vi "WPI_AnalogModuleOpen.vi"(8 "error in (no error)":errorcluster) -> (0 "error out":errorcluster, 3 "AnalogModuleDevRef":T1)   [LabVIEW 2017]
doc: "This software is licensed. Open the labview\\readme\\WPI Robotics Library Open Source License.txt file for more information."
uses:
  <vilib>/Rock Robotics/WPI/AnalogModule/WPI_AnalogModuleDevStatus.ctl
  <vilib>/Rock Robotics/SystemInterfaces/AI/FPGA_AIChannel.ctl
  <vilib>/Rock Robotics/SystemInterfaces/System/FPGA_SystemGet.vi
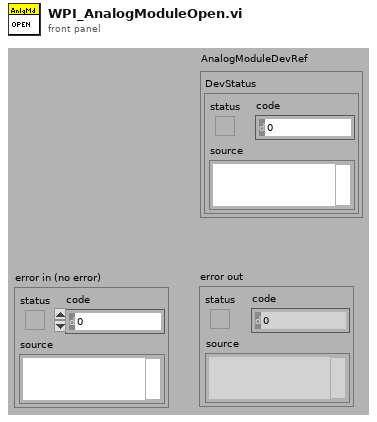
[diagram p1: front panel]
types:
  T1 = typedef "WPI_AnalogModuleDevStatus.ctl" = cluster{"DevStatus":errorcluster}
  T2 = typedef "FPGA_AIDevRef.ctl" = cluster{"DevStatus":errorcluster}
  T3 = typedef "FPGA_AIChannel.ctl" = enum8{"AI 0", "AI 1", "AI 2", "AI 3", "AI MXP 0", "AI MXP 1", "AI MXP 2", "AI MXP 3", "Invalid"}
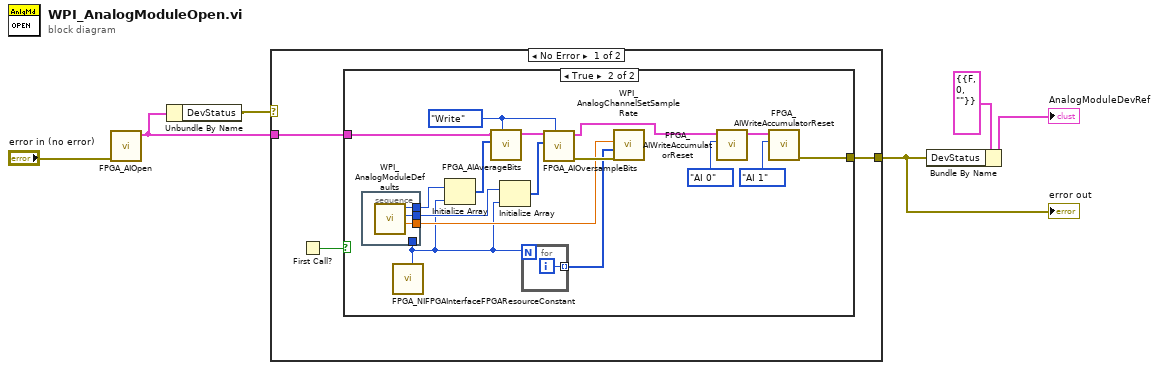
[diagram p0: block diagram]
diagram:
  n1 = call <vilib>:"FPGA_AIOpen.vi"("error in (no error)"="error in (no error)") -> ("AI Reference out"=w3:T2)  [unwired: 2 in, 8 out]
  n2 = Unbundle By Name(w3) -> ("DevStatus"=w4:errorcluster)
  n3 = case shown="No Error" w4 {
    selector: w4 -> [_ w30]
    tunnel: [w9 w30] -> w5
    tunnel: w3 -> [w8 _]
    frame No Error {
      n4 = First Call?() -> (First Call?: T/F=w7:bool)
      n5 = case shown="True" w7 {
        tunnel: [_ w13] -> w9
        tunnel: w8 -> [_ w20]
        frame False {
        }
        frame True {
          w17 = enum16{"Read", "Write"}."Write" ("Task")
          n6 = call <vilib>:"FPGA_NIFPGAInterfaceFPGAResourceConstant.vi"() -> ("NumberOfAIChannels"=w14:u8)  [unwired: 11 out]
          n7 = stacked-sequence {
            tunnel: [w28] -> w24
            tunnel: [w27] -> w22
            tunnel: [w26] -> w15
            tunnel: w14 -> [_]
            frame #0 {
              n8 = call <vilib>:"WPI_AnalogModuleDefaults.vi"() -> ("DEFAULT_SAMPLE_RATE"=w26:dbl, "DEFAULT_OVERSAMPLE_BITS"=w27:u8, "DEFAULT_AVERAGE_BITS"=w28:u8)  [unwired: 9 out]
            }
          }
          n9 = Initialize Array(w24, w14) -> (w23:u8[])
          n10 = call <vilib>:"FPGA_AIAverageBits.vi"("Task"=w17, "AverageBits in"=w23, "AI Reference in"=w20) -> ("AI Reference out"=w25:T2)  [unwired: 1 in, 7 out]
          n11 = Initialize Array(w22, w14) -> (w21:u8[])
          n12 = for {
            N: w14 -> [_]
            tunnel: [w29] -> w18 mode=indexing
            i -> [w29]
          }
          n13 = call <vilib>:"FPGA_AIOversampleBits.vi"("Task"=w17, "OversampleBits in"=w21, "AI Reference in"=w25) -> ("error out"=w19:errorcluster, "AI Reference out"=w16:T2)  [unwired: 1 in, 6 out]
          n14 = call <vilib>:"WPI_AnalogChannelSetSampleRate.vi"("error in (no error)"=w19, "Scan List"=w18, "Samples Per Second (per channel)"=w15) -> ()  [unwired: 2 in, 7 out]
          n15 = call <vilib>:"FPGA_AIWriteAccumulatorReset.vi"("Channel"=FPGA_AIChannel."AI 0", "AI Reference in"=w16) -> ("AI Reference out"=w12:T2)  [unwired: 1 in, 8 out]
          n16 = call <vilib>:"FPGA_AIWriteAccumulatorReset.vi"("Channel"=FPGA_AIChannel."AI 1", "AI Reference in"=w12) -> ("error out"=w13:errorcluster)  [unwired: 1 in, 8 out]
        }
      }
    }
    frame Error {
    }
  }
  "error out" <- w5
  n17 = Bundle By Name(cluster=T1 {"DevStatus"={"status"=FALSE, "code"=0, "source"=""}} ("DevStatus"), "DevStatus"=w5) -> (→"AnalogModuleDevRef":T1)
